vi "Set Custom Device Name.vi"(7 "error in":errorcluster, 9 "name":string, 10 "ni-switch custom device in":T1 format="%.0x") -> (0 "error out":errorcluster, 3 "ni-switch custom device out":T1 format="%.0x")   [LabVIEW 2019, in "NI-SWITCH Scripting.lvlib"]
uses:
  NI-SWITCH Scripting.lvlib
  <vilib>/NI VeriStand/Custom Device API/Custom Device Item Ref.ctl
  <vilib>/NI VeriStand/Custom Device API/Custom Device API.lvlib
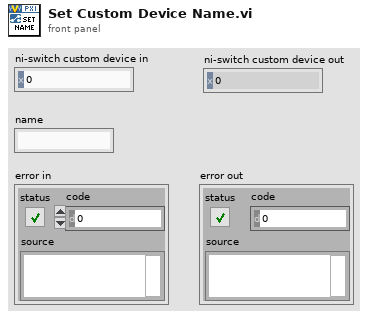
[diagram p1: front panel]
types:
  T1 = typedef "Custom Device API.lvlib/Custom Device Item Ref.ctl" = u64
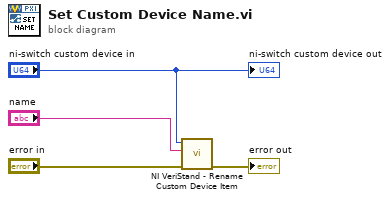
[diagram p0: block diagram]
diagram:
  n1 = call <vilib>:"NI VeriStand - Rename Custom Device Item.vi"("error in (no error)"="error in", "New Name"="name", "Item Ref in"="ni-switch custom device in") -> ("error out"=→"error out":errorcluster)  [unwired: 6 in, 2 out]
  "ni-switch custom device out" <- "ni-switch custom device in"
